vi "Text Field.vi"(8 "error in":errorcluster, 10 "Ctl Refnum":refnum<vi>, 11 "Column Name":string) -> (0 "error out":errorcluster, 3 "Field Configuration":refnum<class "Field Configuration.lvclass">)   [LabVIEW 2020, in "Composed Field Constructors.lvlib"]
uses:
  Composed Field Constructors.lvlib
  Basic Fields/Field Configurations/Field Configuration Class/Field Configuration.lvclass
  Database Libraries/Database Interfaces/Database data type.ctl
  Database Libraries/Database Interfaces.lvlib
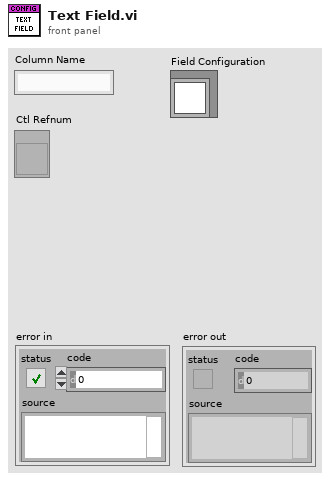
[diagram p1: front panel]
types:
  T1 = typedef "Database Interfaces.lvlib/Database data type.ctl" = enum16{"Undefined", "String", "Long (I32)", "Single (SGL)", "Double (DBL)", "Date/Time", "Binary"}
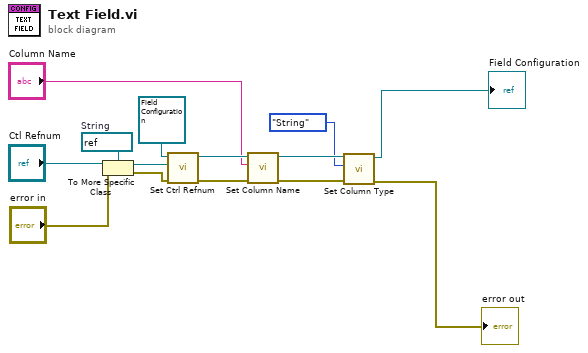
[diagram p0: block diagram]
diagram:
  w8 = refnum<vi> refnum  # String
  n1 = To More Specific Class(target class=w8, reference="Ctl Refnum", error in="error in") -> (specific class reference=w9:refnum<vi>, error out=w7:errorcluster)
  n2 = call-dynamic "Set Ctrl Refnum.vi"("error in (no error)"=w7, "Ctl Refnum"=w9, "Field Configuration in"=refnum<class "Field Configuration.lvclass"> refnum ("Basic Fields.lvlib:Field Configuration.lvclass")) -> ("error out"=w6:errorcluster, "Field Configuration out"=w13:refnum<class "Field Configuration.lvclass">)  [unwired: 7 in]
  n3 = call-dynamic "Set Column Name.vi"("error in (no error)"=w6, "Column Name"="Column Name", "Basic Column Configuration in"=w13) -> ("error out"=w5:errorcluster, "Basic Column Configuration out"=w12:refnum<class "Field Configuration.lvclass">)  [unwired: 7 in]
  n4 = call-dynamic "Set Column Type.vi"("error in (no error)"=w5, "Column Type"=Database_data_type."String", "Basic Column Configuration in"=w12) -> ("error out"=→"error out":errorcluster, "Basic Column Configuration out"=→"Field Configuration":refnum<class "Field Configuration.lvclass">)  [unwired: 7 in]
